vi "AD5781StateMachine.vi"   [LabVIEW 2014]
uses:
  Controls/DacState.ctl
  <vilib>/rvi/Emulation/niFpgaGetClockAttributes.vi
  <vilib>/rvi/Emulation/niFpgaSctlEmulationGetInTimedLoop.vi
  <vilib>/rvi/Emulation/niFpgaEmulationReportErrorSimple.vi
  Code/FPGA SPI_Globals.vi
  <vilib>/rvi/Emulation/niFpgaCriticalErrorInLSC.vi
types:
  T1 = cluster{"SCLK":refnum<k21>, "CS":refnum<k21>, "MOSI":refnum<k21>, "MISO":refnum<k21>}
  T2 = typedef "DacState.ctl" = enum16{"init", "idle", "setVolt", "error"}
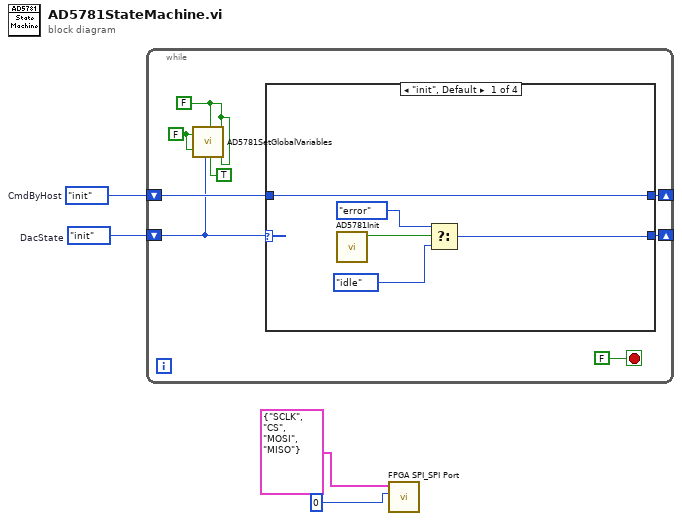
[diagram p0: block diagram]
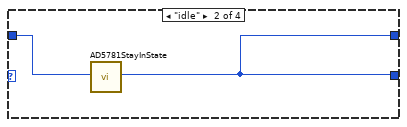
[diagram p2: hidden frame]
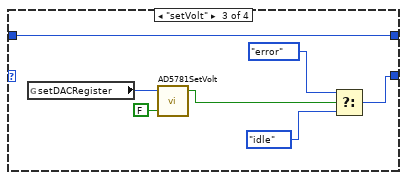
[diagram p3: hidden frame]
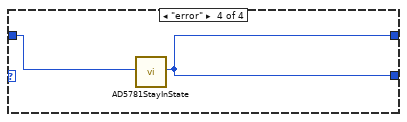
[diagram p4: hidden frame]
diagram:
  w3 = DacState."init"  # CmdByHost
  w4 = DacState."init"  # DacState
  n1 = while {
    shift-right: [w11] -> _
    shift-left: w4 -> [w7]
    shift-right: [w9] -> _
    shift-left: w3 -> [w10]
    stop <- FALSE stop-if-true
    w5 = FALSE ("write DacStateCmdByHost")
    w8 = FALSE ("write actDACRegister")
    n2 = call "AD5781SetGlobalVariables.vi"("write actDACRegister"=w8, "write setDACRegister"=w8, "DacState"=w7, "write DacStateCmdByHost"=w5, "write DacState"=TRUE, "writeSpiGlobals"=w5, "write dac0VRegister"=w5) -> ()  [unwired: 13 in]
    n3 = case shown="\"init\", Default" w7 {
      tunnel: [w17 w18 w22 w27] -> w11
      tunnel: w10 -> [w13 w19 w24 w28]
      tunnel: [w13 w18 w24 w27] -> w9
      frame "init", Default {
        n4 = call "AD5781Init.vi"() -> ("timeOut"=w16:bool)  [unwired: 11 in]
        n5 = Select(t=DacState."error" ("DacState"), s=w16, f=DacState."idle" ("DacState")) -> (s? t:f=w17:T2)
      }
      frame "idle" {
        n6 = call "AD5781StayInState.vi"("lastDacState"=w19) -> ("newDacState"=w18:T2)  [unwired: 18 in]
      }
      frame "setVolt" {
        n7 = global read "FPGA SPI_Globals.vi" "setDACRegister"() -> (w26:u32)
        n8 = call "AD5781SetVolt.vi"("Send"=FALSE, "SetVolt"=w26) -> ("timedOut"=w23:bool)  [unwired: 1 in, 2 out]
        n9 = Select(t=DacState."error" ("DacState"), s=w23, f=DacState."idle" ("DacState")) -> (s? t:f=w22:T2)
      }
      frame "error" {
        n10 = call "AD5781StayInState.vi"("lastDacState"=w28) -> ("newDacState"=w27:T2)  [unwired: 18 in]
      }
    }
  }
  n11 = call "FPGA SPI_SPI Port.vi"("Port"=i8 0, "FPGA IO"=T1 {"SCLK"="SCLK", "CS"="CS", "MOSI"="MOSI", "MISO"="MISO"}) -> ()  [unwired: 10 in]
